vi "SPI write many.vi"(4 "values":u8[](array[numeric]), 6 "addresses":u8[](array[numeric]), 8 "error in (no error)":errorcluster, 10 "spi configuration in":T2, 11 "Device ref in":T1) -> (0 "error out":errorcluster, 2 "spi configuration out":T2, 3 "Device ref out":T1)   [LabVIEW 2013]
uses:
  <vilib>/ni845x/ni845x.llb/ni845xSpiConfiguration.ctl
  <vilib>/ni845x/ni845x.llb/ni845xControl.ctl
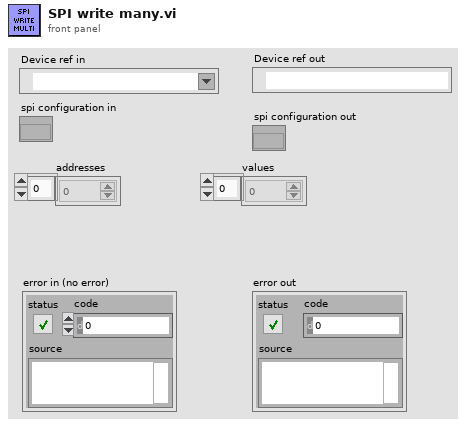
[diagram p1: front panel]
types:
  T1 = typedef "ni845xControl.ctl" = refnum<k21>
  T2 = typedef "ni845xSpiConfiguration.ctl" = refnum<k20>
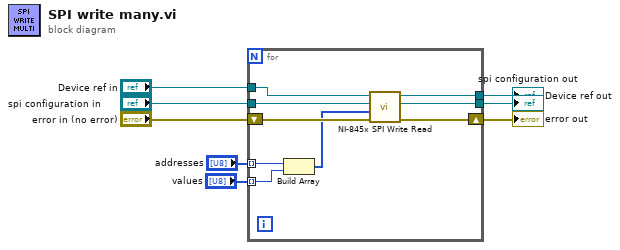
[diagram p0: block diagram]
diagram:
  n1 = for {
    tunnel: [w16] -> w7
    tunnel: [w15] -> w6
    tunnel: "spi configuration in" -> [w13]
    tunnel: "Device ref in" -> [w12]
    tunnel: "addresses" -> [w11] mode=indexing
    tunnel: "values" -> [w10] mode=indexing
    shift-right: [w17] -> w8
    shift-left: "error in (no error)" -> [w14]
    n2 = Build Array(w11, w10) -> (w9:u8[])
    n3 = call <vilib>:"NI-845x SPI Write Read.vi"("error in (no error)"=w14, "write data"=w9, "spi configuration in"=w13, "device reference in"=w12) -> ("error out"=w17:errorcluster, "spi configuration out"=w16:T2, "device reference out"=w15:T1)  [unwired: 4 in, 1 out]
  }
  "error out" <- w8
  "spi configuration out" <- w7
  "Device ref out" <- w6
